vi "Config Limit Setting.vi"(0 "VISA resource name":refnum<visa-resource-name>, 5 "Source Setting (T:Voltage)":bool=TRUE, 7 "High Limit (1.00E+3)":dbl=1000.0 format="%^.2e", 11 "error in (no error)":errorcluster) -> (4 "VISA resource name out":refnum<visa-resource-name>, 15 "error out":errorcluster)   [LabVIEW 2020, in "Stanford Research PS300 Series.lvlib"]
doc: "This VI configures the output source and then specifies the highest output value for that source.\n\nIf having problems setting output voltage, voltage limit, or current limit, try negating your voltage or current value."
uses:
  Stanford Research PS300 Series.lvlib
panel:
  # "Voltage\nCurrent"
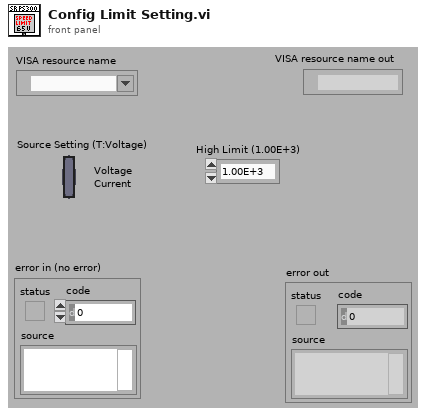
[diagram p1: front panel]
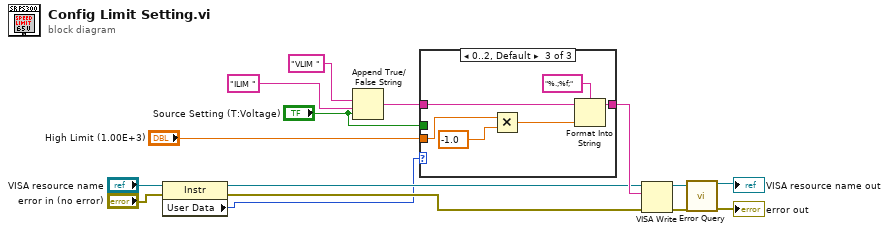
[diagram p0: block diagram]
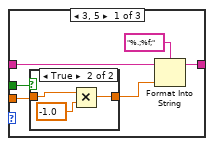
[diagram p2: hidden frame]
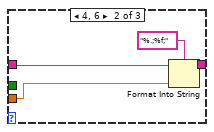
[diagram p4: hidden frame]
diagram:
  n1 = property class="Instr"(reference="VISA resource name", error in="error in (no error)") -> (reference out=w4:refnum<visa-resource-name>, error out=w3:errorcluster, "User Data"=w2:u32)
  n2 = Append True/False String(1:"Source Setting (T:Voltage)", 2:"ILIM " ("false string"), 3:"VLIM " ("true string")) -> (0:w15:string)  [unwired: 1 in]
  n3 = case shown="0..2, Default" w2 {
    tunnel: w15 -> [w19 w27 w35]
    tunnel: [w18 w26 w34] -> w14
    tunnel: "High Limit (1.00E+3)" -> [w17 w29 w30]
    tunnel: "Source Setting (T:Voltage)" -> [w16 _ _]
    frame 3, 5 {
      n4 = case shown="True" w16 {
        tunnel: [w22 w24] -> w21
        tunnel: w17 -> [w22 w23]
        frame False {
        }
        frame True {
          n5 = Multiply(x=w23, y=-1.0) -> (x*y=w24:dbl)
        }
      }
      n6 = Format Into String(format string="%.;%f;", initial string=w19, w21) -> (resulting string=w18:string)  [unwired: 1 in, 1 out]
    }
    frame 4, 6 {
      n7 = Format Into String(format string="%.;%f;", initial string=w27, w29) -> (resulting string=w26:string)  [unwired: 1 in, 1 out]
    }
    frame 0..2, Default {
      n8 = Multiply(x=w30, y=-1.0) -> (x*y=w31:dbl)
      n9 = Format Into String(format string="%.;%f;", initial string=w35, w31) -> (resulting string=w34:string)  [unwired: 1 in, 1 out]
    }
  }
  n10 = VISA Write(VISA resource name=w4, write buffer=w14, error in (no error)=w3) -> (VISA resource name out=w11:refnum<visa-resource-name>, error out=w10:errorcluster)  [unwired: 1 out]
  n11 = call "Error Query.vi"("VISA resource name"=w11, "error in (no error)"=w10) -> ("VISA resource name out"=→"VISA resource name out":refnum<visa-resource-name>, "error out"=→"error out":errorcluster)  [unwired: 10 in, 2 out]
